vi "Email Handler (RT).vi"   [LabVIEW 2019]
types:
  T1 = cluster{"ArmedAddresses":i32[], "Tracker":i32, "EmailArray":i32[], "Armed":bool, "Inform":string, "Alarm":bool}
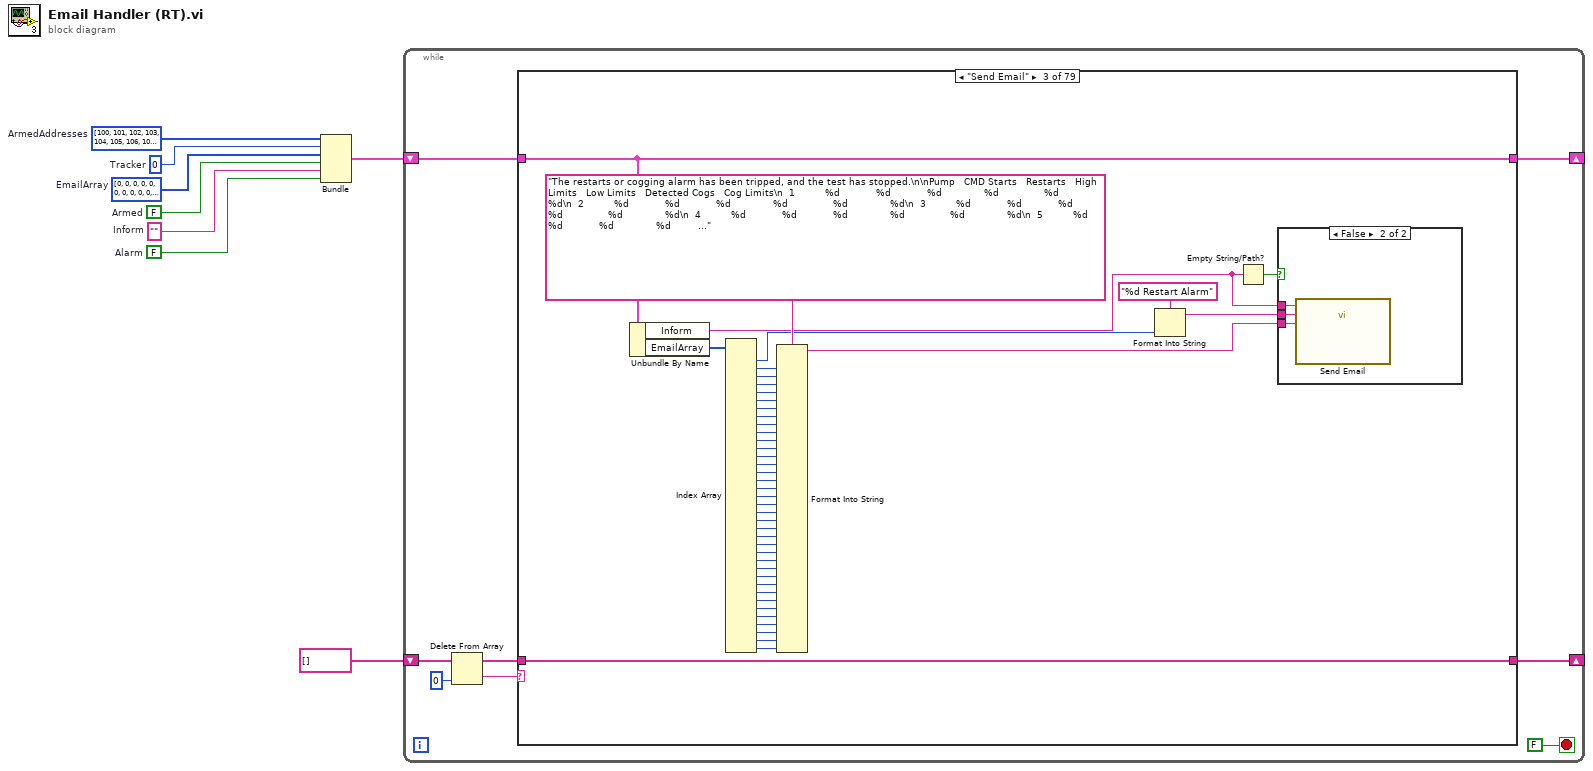
[diagram p0: block diagram]
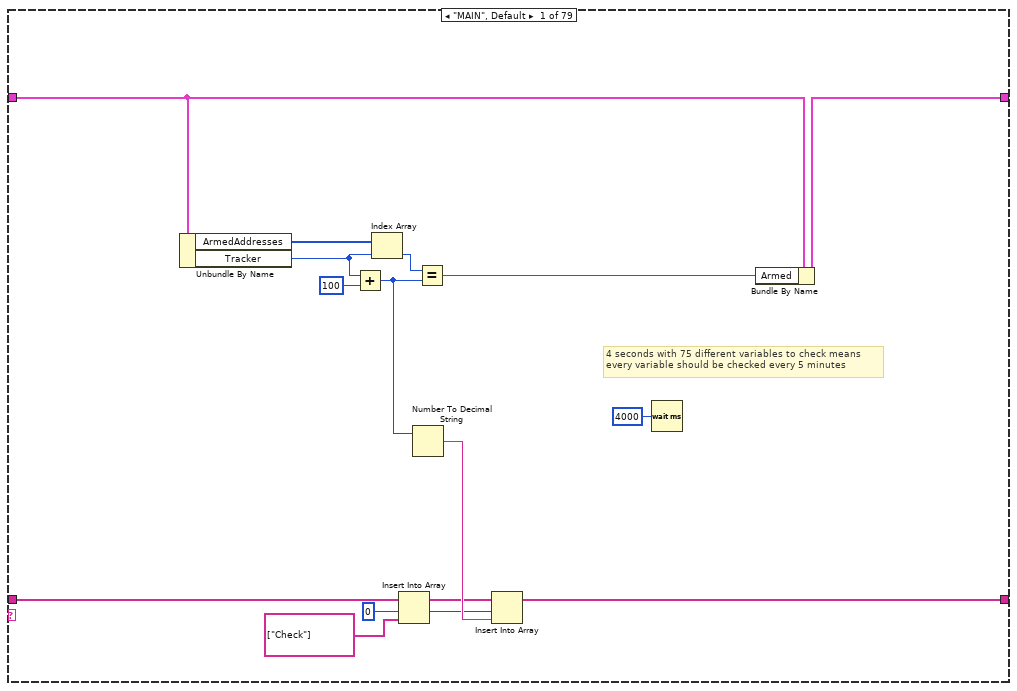
[diagram p2: hidden frame]
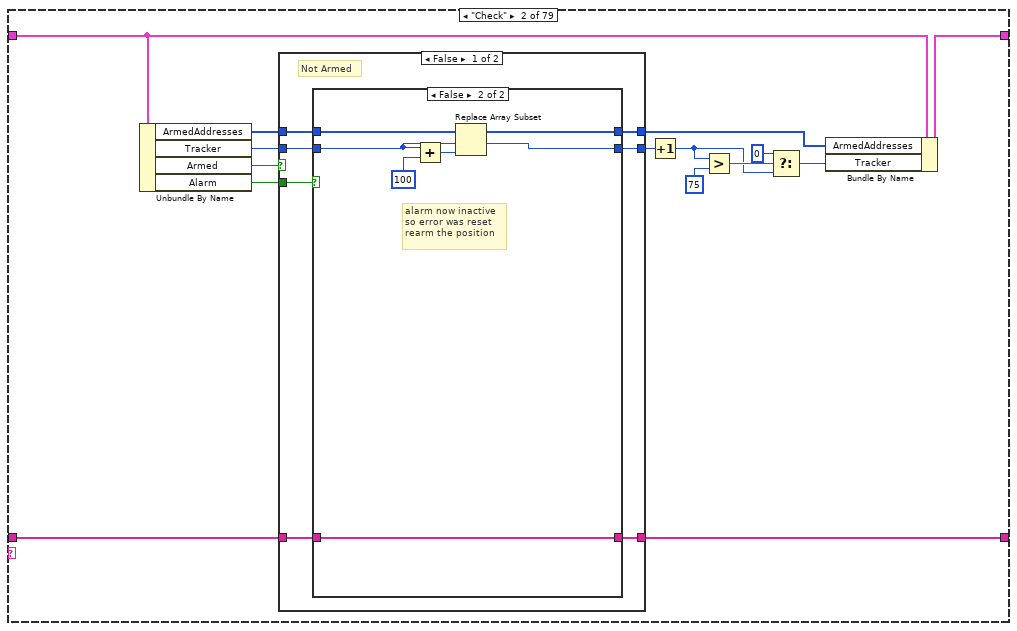
[diagram p3: hidden frame]
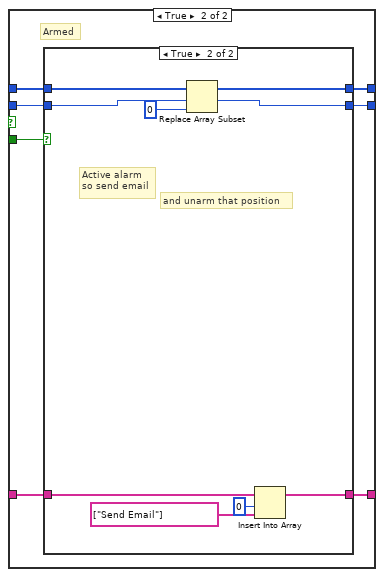
[diagram p5: hidden frame]
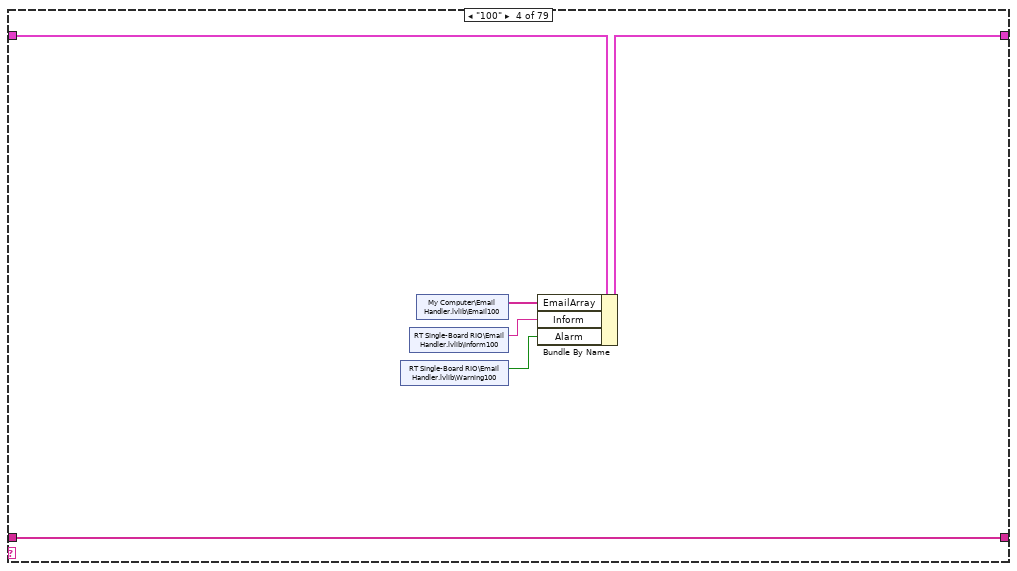
[diagram p8: hidden frame]
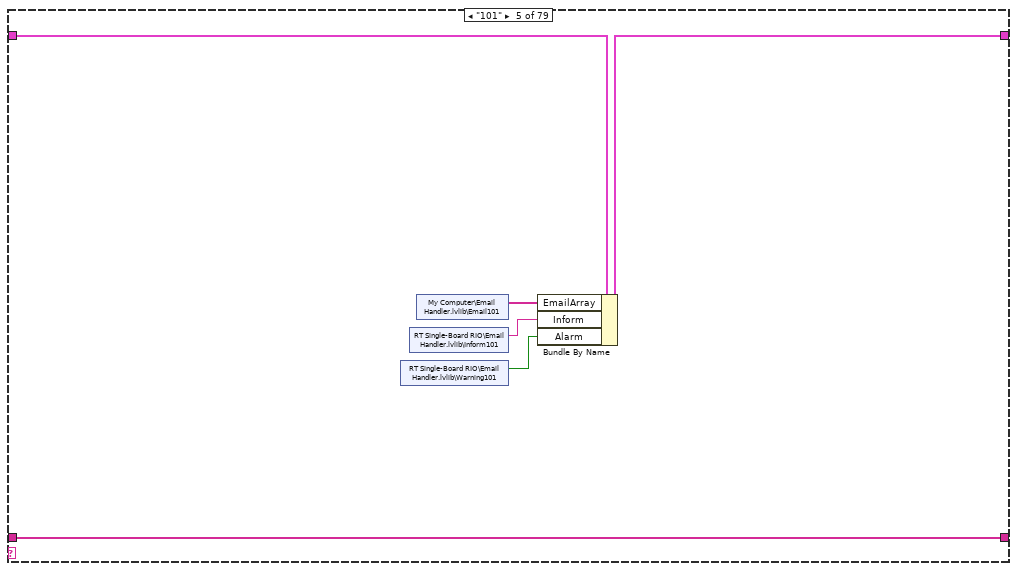
[diagram p9: hidden frame]
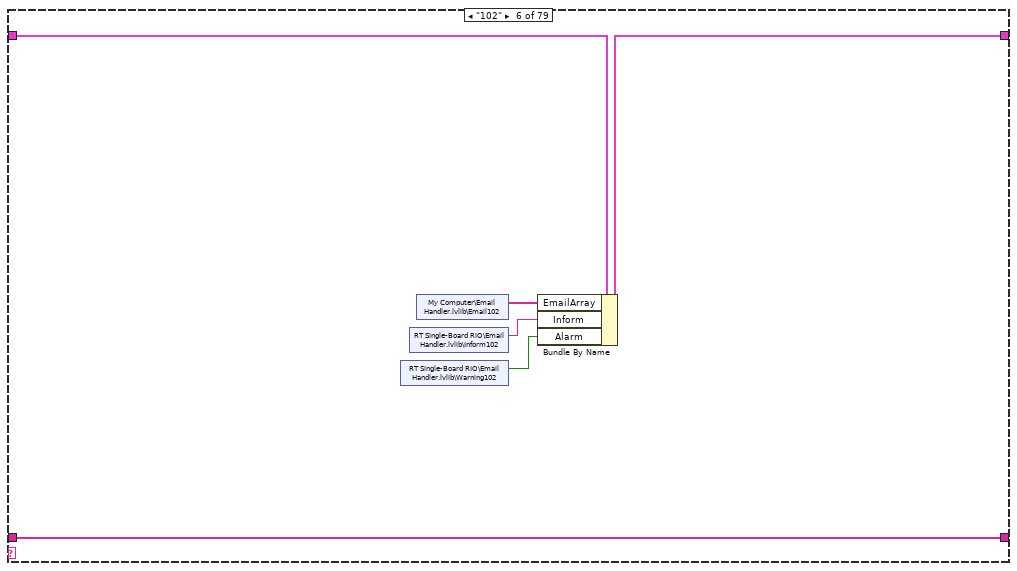
[diagram p10: hidden frame]
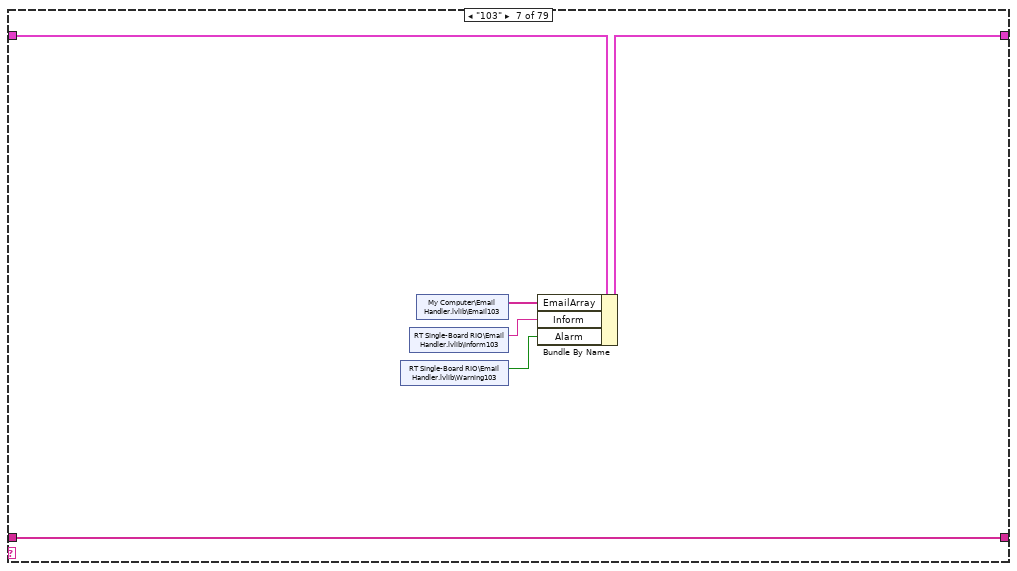
[diagram p11: hidden frame]
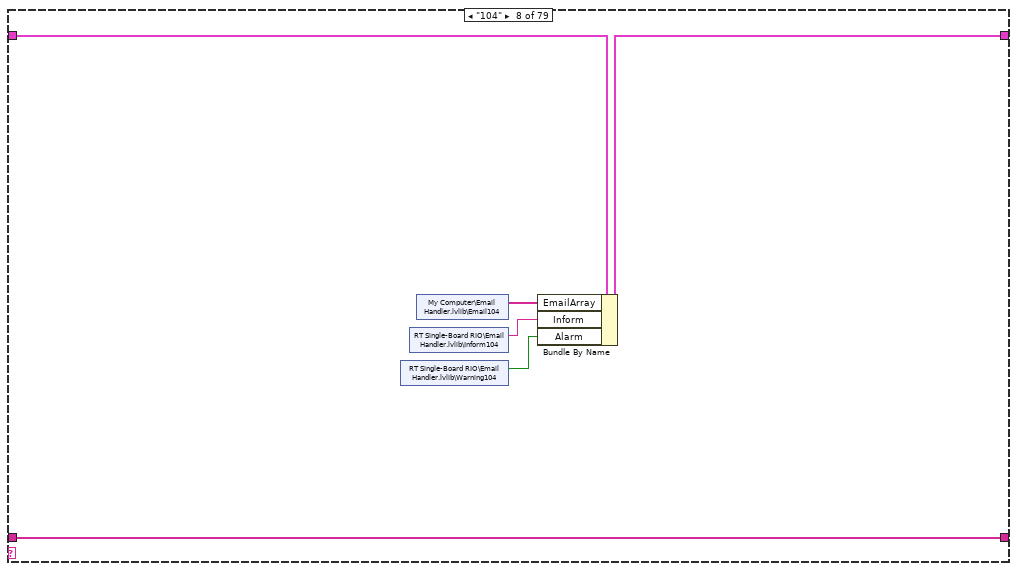
[diagram p12: hidden frame]
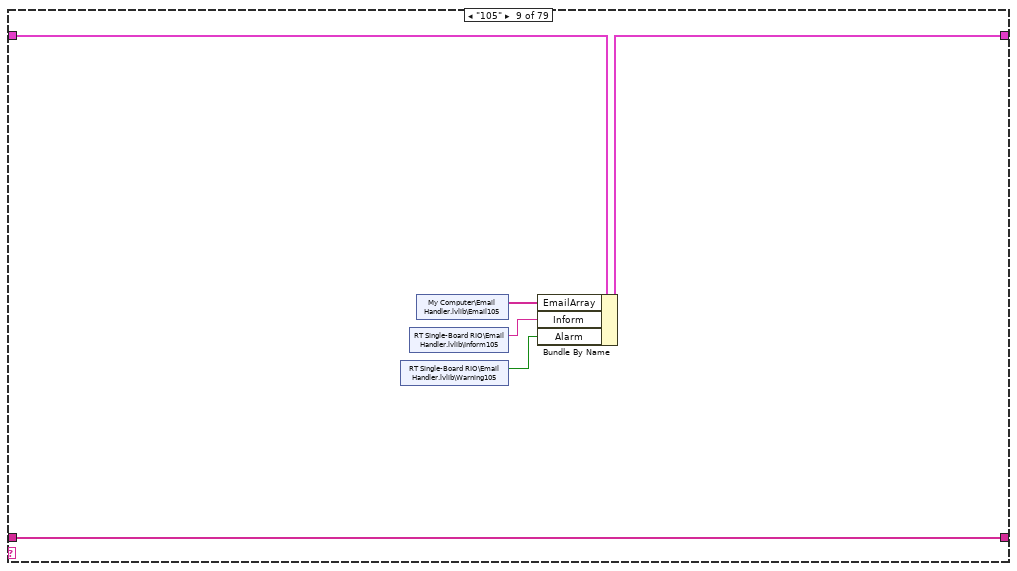
[diagram p13: hidden frame]
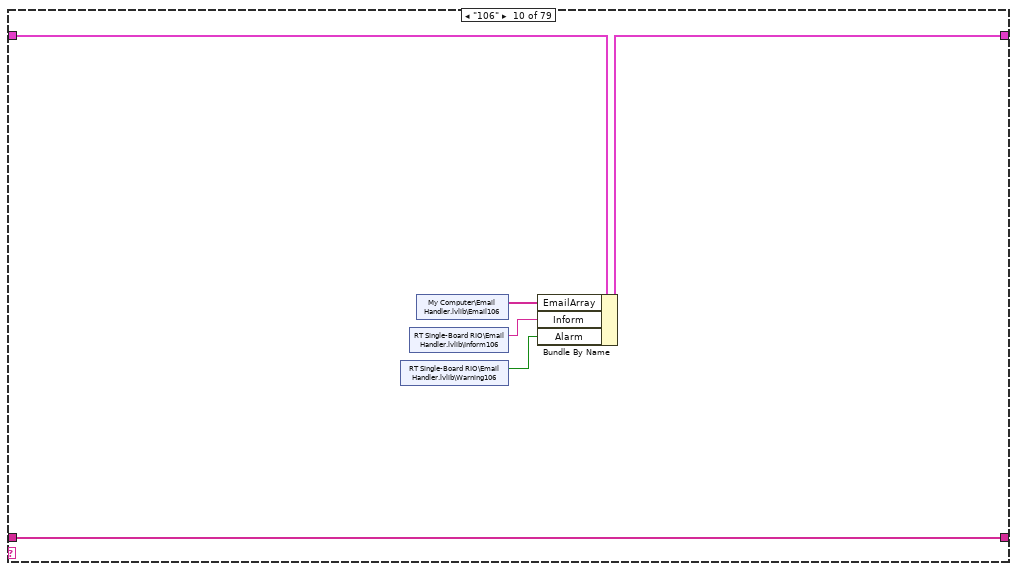
[diagram p14: hidden frame]
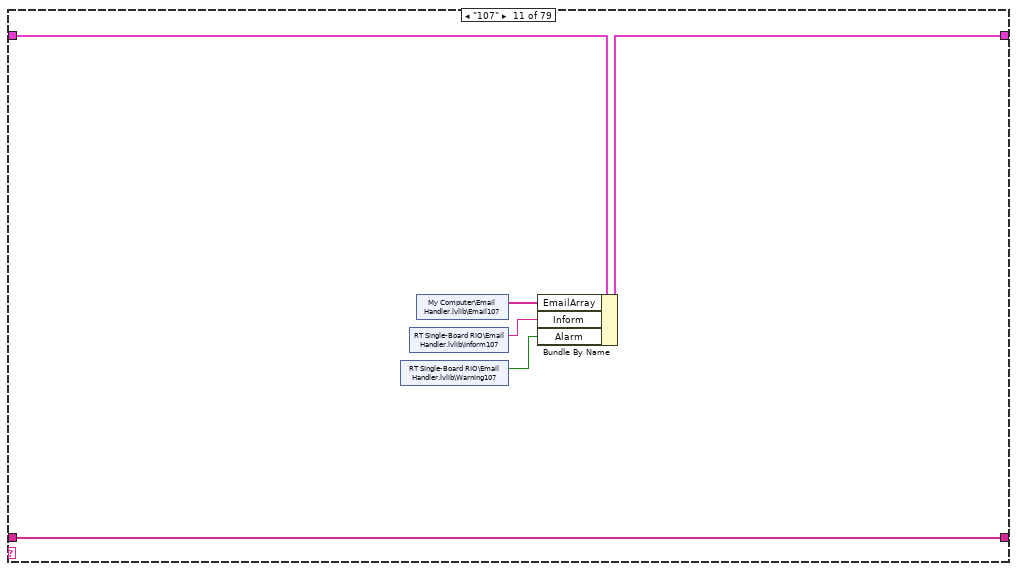
[diagram p15: hidden frame]
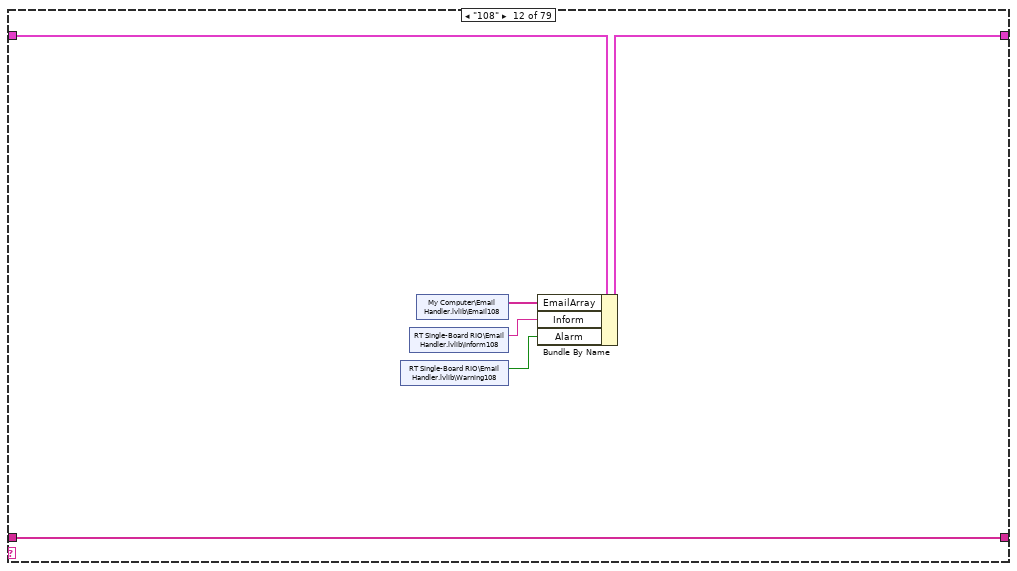
[diagram p16: hidden frame]
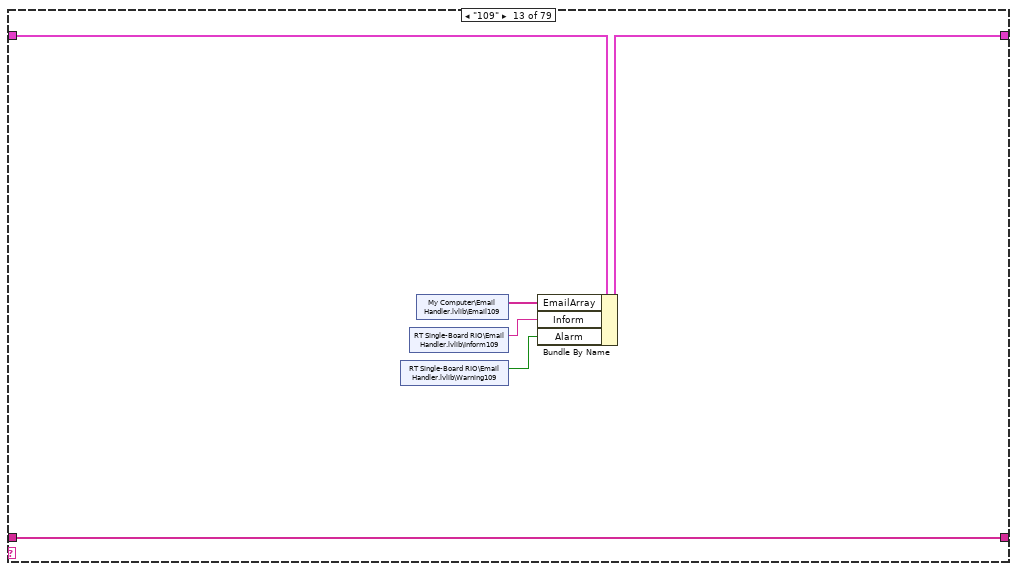
[diagram p17: hidden frame]
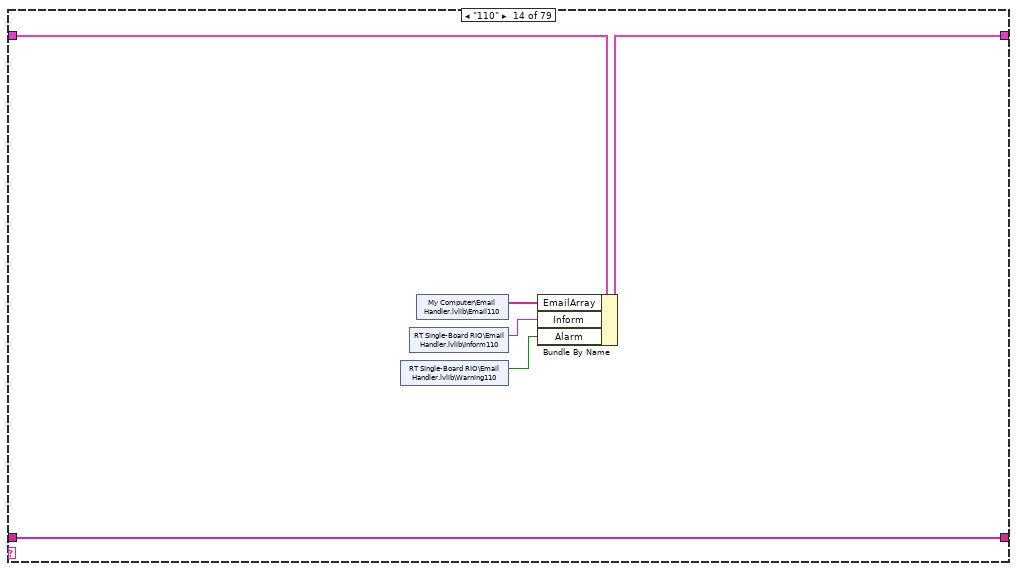
[diagram p18: hidden frame]
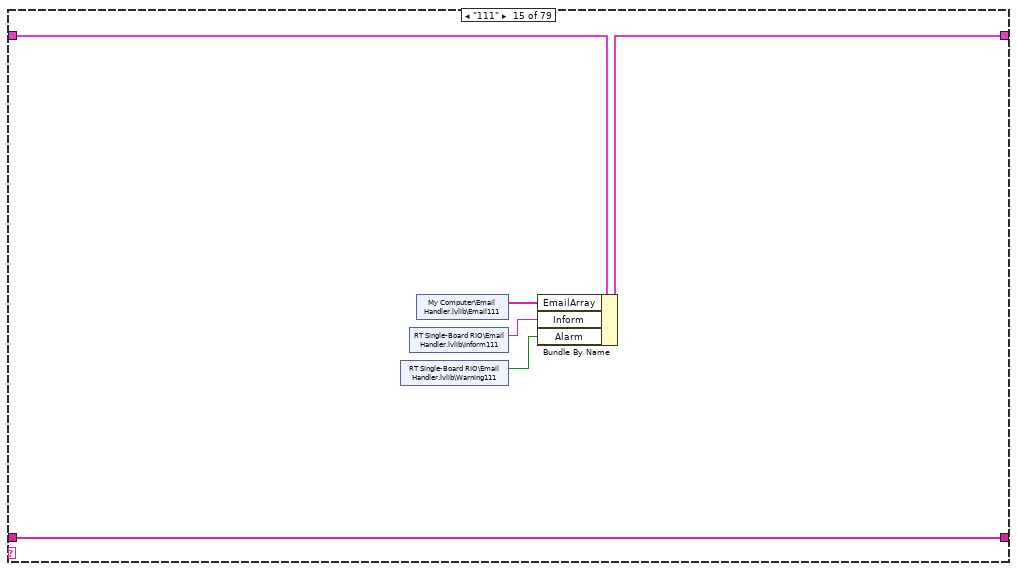
[diagram p19: hidden frame]
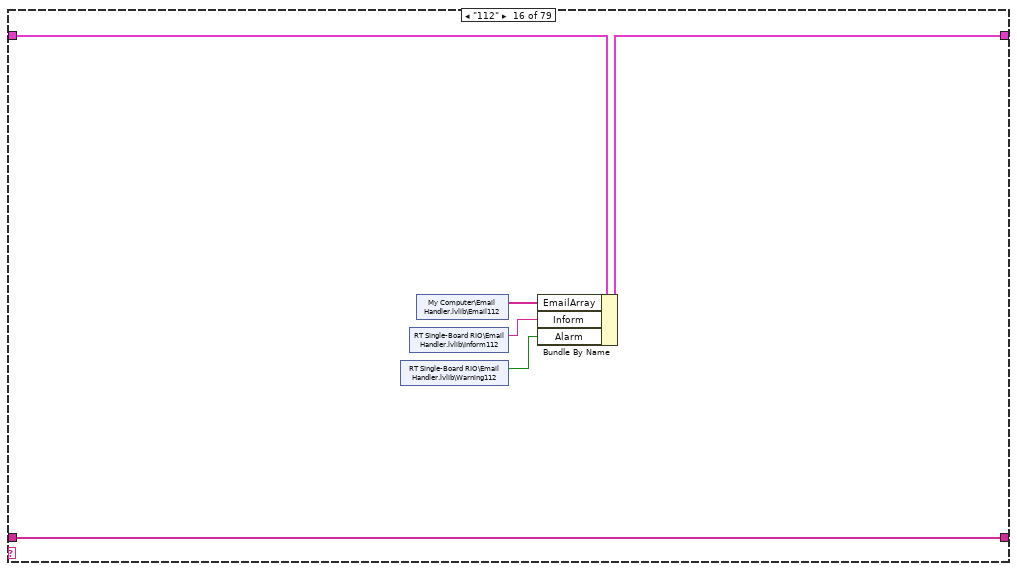
[diagram p20: hidden frame]
diagram:
  w1 = FALSE  # Alarm
  w2 = ""  # Inform
  w3 = FALSE  # Armed
  w4 = i32[] [0, 0, 0, 0, 0, 0, 0, 0, 0, 0, 0, 0, 0, 0, 0, 0, 0, 0, 0, 0, 0, 0, 0, 0, 0, 0, 0, 0, 0, 0, 0, 0, 0, 0, 0, 0, 0]  # EmailArray
  w6 = i32[] [100, 101, 102, 103, 104, 105, 106, 107, 108, 109, 110, 111, 112, 113, 114, 115, 116, 117, 118, 119, 120, 121, 122, 123, 124, 125, 126, 127, 128, 129, 130, 131, 132, 133, 134, 135, 136, 137, 138, 139, 140, 141, 142, 143, 144, 145, 146, 147, 148, 149, 150, 151, 152, 153, 154, 155, 156, 157, 158, 159, 160, 161, 162, 163, 164, 165, 166, 167, 168, 169, 170, 171, 172, 173, 174, 175]  # ArmedAddresses
  w8 = 0  # Tracker
  n1 = Bundle("ArmedAddresses"=w6, "Tracker"=w8, "EmailArray"=w4, "Armed"=w3, "Inform"=w2, "Alarm"=w1) -> (w7:T1)  [unwired: 1 in]
  n2 = while {
    shift-right: [w9] -> _
    shift-left: w7 -> [w15]
    shift-right: [w10] -> _
    shift-left: string[] [] -> [w14]
    stop <- FALSE stop-if-true
    n3 = Delete From Array(array=w14, index=0) -> (deleted portion=w12:string, array with subset deleted=w11:string[])  [unwired: 1 in]
    n4 = case shown="\"Send Email\"" w12 {
      tunnel: w15 -> [w29 w41 w125 w134 w140 w146 w152 w158 w164 w170 w176 w182 w188 w194 w200 w206 w212 w218 w224 w230 w236 w242 w248 w254 w260 w266 w272 w278 w284 w290 w296 w302 w308 w314 w320 w326 w332 w338 w344 w350 w356 w362 w368 w374 w380 w386 w392 w398 w404 w410 w416 w422 w428 w434 w440 w446 w452 w458 w464 w470 w476 w482 w488 w494 w500 w506 w512 w518 w524 w530 w536 w542 w548 w554 w560 w566 w572 w578 w584]
      tunnel: w11 -> [w21 w38 w126 w135 w141 w147 w153 w159 w165 w171 w177 w183 w189 w195 w201 w207 w213 w219 w225 w231 w237 w243 w249 w255 w261 w267 w273 w279 w285 w291 w297 w303 w309 w315 w321 w327 w333 w339 w345 w351 w357 w363 w369 w375 w381 w387 w393 w399 w405 w411 w417 w423 w429 w435 w441 w447 w453 w459 w465 w471 w477 w483 w489 w495 w501 w507 w513 w519 w525 w531 w537 w543 w549 w555 w561 w567 w573 w579 w585]
      tunnel: [w23 w35 w126 w135 w141 w147 w153 w159 w165 w171 w177 w183 w189 w195 w201 w207 w213 w219 w225 w231 w237 w243 w249 w255 w261 w267 w273 w279 w285 w291 w297 w303 w309 w315 w321 w327 w333 w339 w345 w351 w357 w363 w369 w375 w381 w387 w393 w399 w405 w411 w417 w423 w429 w435 w441 w447 w453 w459 w465 w471 w477 w483 w489 w495 w501 w507 w513 w519 w525 w531 w537 w543 w549 w555 w561 w567 w573 w579 w585] -> w10
      tunnel: [w28 w40 w125 w133 w139 w145 w151 w157 w163 w169 w175 w181 w187 w193 w199 w205 w211 w217 w223 w229 w235 w241 w247 w253 w259 w265 w271 w277 w283 w289 w295 w301 w307 w313 w319 w325 w331 w337 w343 w349 w355 w361 w367 w373 w379 w385 w391 w397 w403 w409 w415 w421 w427 w433 w439 w445 w451 w457 w463 w469 w475 w481 w487 w493 w499 w505 w511 w517 w523 w529 w535 w541 w547 w553 w559 w565 w571 w577 w583] -> w9
      frame "MAIN", Default {
        w19 = 0 ("index")
        # "4 seconds with 75 different variables to check means\nevery variable should be checked every 5 minutes"
        n5 = Unbundle By Name(w29) -> ("ArmedAddresses"=w30:i32[], "Tracker"=w17:i32)
        n6 = Add(x=w17, y=100) -> (x+y=w25:i32)
        n7 = Index Array(array=w30, index=w17) -> (element=w26:i32)
        n8 = Insert Into Array(array=w21, index=w19, new element=string[] ["Check"]) -> (w20:string[])
        n9 = Number To Decimal String(number=w25) -> (decimal integer string=w24:string)  [unwired: 1 in]
        n10 = Equal?(x=w26, y=w25) -> (x = y?=w22:bool)
        n11 = Insert Into Array(array=w20, index=w19, new element=w24) -> (w23:string[])
        n12 = Wait (ms)(milliseconds to wait=u32 4000) -> ()  [unwired: 1 out]
        n13 = Bundle By Name(cluster=w29, "Armed"=w22) -> (w28:T1)
      }
      frame "Check" {
        n14 = Unbundle By Name(w41) -> ("ArmedAddresses"=w34:i32[], "Tracker"=w37:i32, "Armed"=w39:bool, "Alarm"=w32:bool)
        n15 = case shown="False" w39 {
          tunnel: w38 -> [w53 w69]
          tunnel: w37 -> [w50 w66]
          tunnel: [w47 w63] -> w36
          tunnel: w32 -> [w49 w67]
          tunnel: [w52 w68] -> w35
          tunnel: w34 -> [w51 w65]
          tunnel: [w48 w64] -> w33
          frame False {
            # "Not Armed"
            n16 = case shown="False" w49 {
              tunnel: w53 -> [w54 w57]
              tunnel: [w54 w57] -> w52
              tunnel: w50 -> [w55 w60]
              tunnel: w51 -> [w56 w62]
              tunnel: [w56 w61] -> w48
              tunnel: [w55 w60] -> w47
              frame True {
                # "Alarm still active\nerror has not been reset\nleave unarmed"
              }
              frame False {
                # "alarm now inactive\nso error was reset\nrearm the position"
                n17 = Add(x=w60, y=100) -> (x+y=w59:i32)
                n18 = Replace Array Subset(array=w62, new element=w59, index=w60) -> (w61:i32[])
              }
            }
          }
          frame True {
            # "Armed"
            n19 = case shown="True" w67 {
              tunnel: w69 -> [w70 w80]
              tunnel: [w70 w79] -> w68
              tunnel: w66 -> [w71 w74]
              tunnel: w65 -> [w72 w76]
              tunnel: [w72 w75] -> w64
              tunnel: [w71 w74] -> w63
              frame False {
                # "No Alarm"
              }
              frame True {
                # "and unarm that position"
                # "Active alarm\nso send email"
                n20 = Replace Array Subset(array=w76, new element=0, index=w74) -> (w75:i32[])
                n21 = Insert Into Array(array=w80, index=0, new element=string[] ["Send Email"]) -> (w79:string[])
              }
            }
          }
        }
        n22 = Increment(x=w36) -> (x+1=w43:i32)
        n23 = Greater?(x=w43, y=75) -> (0:w45:bool)
        n24 = Select(t=0, s=w45, f=w43) -> (s? t:f=w42:i32)
        n25 = Bundle By Name(cluster=w41, "ArmedAddresses"=w33, "Tracker"=w42) -> (w40:T1)
      }
      frame "Send Email" {
        n26 = Unbundle By Name(w125) -> ("Inform"=w82:string, "EmailArray"=w96:i32[])
        n27 = Index Array(array=w96) -> (element #1=w83:i32, element #2=w100:i32, element #3=w101:i32, element #4=w102:i32, element #5=w103:i32, element #6=w104:i32, element #7=w105:i32, element #8=w106:i32, element #9=w107:i32, element #10=w108:i32, element #11=w109:i32, element #12=w110:i32, element #13=w111:i32, element #14=w114:i32, element #15=w113:i32, element #16=w115:i32, element #17=w116:i32, element #18=w117:i32, element #19=w118:i32, element #20=w119:i32, element #21=w120:i32, element #22=w121:i32, element #23=w122:i32, element #24=w123:i32, element #25=w124:i32, element #26=w95:i32, element #27=w94:i32, element #28=w93:i32, element #29=w92:i32, element #30=w91:i32, element #31=w90:i32, element #32=w89:i32, element #33=w88:i32, element #34=w87:i32, element #35=w86:i32, element #36=w85:i32, element #37=w84:i32)  [unwired: 37 in]
        n28 = Format Into String(format string="The restarts or cogging alarm has been tripped, and the test has stopped.\n\nPump   CMD Starts   Restarts   High Limits   Low Limits   Detected Cogs   Cog Limits\n  1          %d            %d            %d              %d               %d              %d\n  2          %d            %d            %d              %d               %d              %d\n  3          %d            %d            %d              %d               %d              %d\n  4          %d            %d            %d              %d               %d              %d\n  5          %d            %d            %d              %d               %d              %d\n  6          %d            %d            %d              %d               %d              %d" ("Message"), w100, w101, w102, w103, w104, w105, w106, w107, w108, w109, w110, w111, w114, w113, w115, w116, w117, w118, w119, w120, w121, w122, w123, w124, w95, w94, w93, w92, w91, w90, w89, w88, w87, w86, w85, w84) -> (resulting string=w112:string)  [unwired: 2 in, 1 out]
        n29 = Format Into String(format string="%d Restart Alarm", w83) -> (resulting string=w98:string)  [unwired: 2 in, 1 out]
        n30 = Empty String/Path?(string/path=w82) -> (empty?=w81:bool)
        n31 = case shown="False" w81 {
          tunnel: w112 -> [_ w129]
          tunnel: w98 -> [_ w128]
          tunnel: w82 -> [_ w127]
          frame True {
          }
          frame False {
            n32 = call "Send Email"("Message"=w129, "Subject"=w128, "Recipients"=w127) -> ()  [unwired: 8 in, 1 out]
          }
        }
      }
      frame "100" {
        n33 = shared-variable "RT Single-Board RIO\\Email Handler.lvlib\\Warning100"() -> (w130:bool)  [unwired: 1 in, 1 out]
        n34 = shared-variable "RT Single-Board RIO\\Email Handler.lvlib\\Inform100"() -> (w131:string)  [unwired: 1 in, 1 out]
        n35 = shared-variable "My Computer\\Email Handler.lvlib\\Email100"() -> (w132:string[])  [unwired: 1 in, 1 out]
        n36 = Bundle By Name(cluster=w134, "EmailArray"=w132, "Inform"=w131, "Alarm"=w130) -> (w133:T1)
      }
      frame "101" {
        n37 = shared-variable "RT Single-Board RIO\\Email Handler.lvlib\\Warning101"() -> (w136:bool)  [unwired: 1 in, 1 out]
        n38 = shared-variable "RT Single-Board RIO\\Email Handler.lvlib\\Inform101"() -> (w137:string)  [unwired: 1 in, 1 out]
        n39 = shared-variable "My Computer\\Email Handler.lvlib\\Email101"() -> (w138:string[])  [unwired: 1 in, 1 out]
        n40 = Bundle By Name(cluster=w140, "EmailArray"=w138, "Inform"=w137, "Alarm"=w136) -> (w139:T1)
      }
      frame "102" {
        n41 = shared-variable "RT Single-Board RIO\\Email Handler.lvlib\\Warning102"() -> (w142:bool)  [unwired: 1 in, 1 out]
        n42 = shared-variable "RT Single-Board RIO\\Email Handler.lvlib\\Inform102"() -> (w143:string)  [unwired: 1 in, 1 out]
        n43 = shared-variable "My Computer\\Email Handler.lvlib\\Email102"() -> (w144:string[])  [unwired: 1 in, 1 out]
        n44 = Bundle By Name(cluster=w146, "EmailArray"=w144, "Inform"=w143, "Alarm"=w142) -> (w145:T1)
      }
      frame "103" {
        n45 = shared-variable "RT Single-Board RIO\\Email Handler.lvlib\\Warning103"() -> (w148:bool)  [unwired: 1 in, 1 out]
        n46 = shared-variable "RT Single-Board RIO\\Email Handler.lvlib\\Inform103"() -> (w149:string)  [unwired: 1 in, 1 out]
        n47 = shared-variable "My Computer\\Email Handler.lvlib\\Email103"() -> (w150:string[])  [unwired: 1 in, 1 out]
        n48 = Bundle By Name(cluster=w152, "EmailArray"=w150, "Inform"=w149, "Alarm"=w148) -> (w151:T1)
      }
      frame "104" {
        n49 = shared-variable "RT Single-Board RIO\\Email Handler.lvlib\\Warning104"() -> (w154:bool)  [unwired: 1 in, 1 out]
        n50 = shared-variable "RT Single-Board RIO\\Email Handler.lvlib\\Inform104"() -> (w155:string)  [unwired: 1 in, 1 out]
        n51 = shared-variable "My Computer\\Email Handler.lvlib\\Email104"() -> (w156:string[])  [unwired: 1 in, 1 out]
        n52 = Bundle By Name(cluster=w158, "EmailArray"=w156, "Inform"=w155, "Alarm"=w154) -> (w157:T1)
      }
      frame "105" {
        n53 = shared-variable "RT Single-Board RIO\\Email Handler.lvlib\\Warning105"() -> (w160:bool)  [unwired: 1 in, 1 out]
        n54 = shared-variable "RT Single-Board RIO\\Email Handler.lvlib\\Inform105"() -> (w161:string)  [unwired: 1 in, 1 out]
        n55 = shared-variable "My Computer\\Email Handler.lvlib\\Email105"() -> (w162:string[])  [unwired: 1 in, 1 out]
        n56 = Bundle By Name(cluster=w164, "EmailArray"=w162, "Inform"=w161, "Alarm"=w160) -> (w163:T1)
      }
      frame "106" {
        n57 = shared-variable "RT Single-Board RIO\\Email Handler.lvlib\\Warning106"() -> (w166:bool)  [unwired: 1 in, 1 out]
        n58 = shared-variable "RT Single-Board RIO\\Email Handler.lvlib\\Inform106"() -> (w167:string)  [unwired: 1 in, 1 out]
        n59 = shared-variable "My Computer\\Email Handler.lvlib\\Email106"() -> (w168:string[])  [unwired: 1 in, 1 out]
        n60 = Bundle By Name(cluster=w170, "EmailArray"=w168, "Inform"=w167, "Alarm"=w166) -> (w169:T1)
      }
      frame "107" {
        n61 = shared-variable "RT Single-Board RIO\\Email Handler.lvlib\\Warning107"() -> (w172:bool)  [unwired: 1 in, 1 out]
        n62 = shared-variable "RT Single-Board RIO\\Email Handler.lvlib\\Inform107"() -> (w173:string)  [unwired: 1 in, 1 out]
        n63 = shared-variable "My Computer\\Email Handler.lvlib\\Email107"() -> (w174:string[])  [unwired: 1 in, 1 out]
        n64 = Bundle By Name(cluster=w176, "EmailArray"=w174, "Inform"=w173, "Alarm"=w172) -> (w175:T1)
      }
      frame "108" {
        n65 = shared-variable "RT Single-Board RIO\\Email Handler.lvlib\\Warning108"() -> (w178:bool)  [unwired: 1 in, 1 out]
        n66 = shared-variable "RT Single-Board RIO\\Email Handler.lvlib\\Inform108"() -> (w179:string)  [unwired: 1 in, 1 out]
        n67 = shared-variable "My Computer\\Email Handler.lvlib\\Email108"() -> (w180:string[])  [unwired: 1 in, 1 out]
        n68 = Bundle By Name(cluster=w182, "EmailArray"=w180, "Inform"=w179, "Alarm"=w178) -> (w181:T1)
      }
      frame "109" {
        n69 = shared-variable "RT Single-Board RIO\\Email Handler.lvlib\\Warning109"() -> (w184:bool)  [unwired: 1 in, 1 out]
        n70 = shared-variable "RT Single-Board RIO\\Email Handler.lvlib\\Inform109"() -> (w185:string)  [unwired: 1 in, 1 out]
        n71 = shared-variable "My Computer\\Email Handler.lvlib\\Email109"() -> (w186:string[])  [unwired: 1 in, 1 out]
        n72 = Bundle By Name(cluster=w188, "EmailArray"=w186, "Inform"=w185, "Alarm"=w184) -> (w187:T1)
      }
      frame "110" {
        n73 = shared-variable "RT Single-Board RIO\\Email Handler.lvlib\\Warning110"() -> (w190:bool)  [unwired: 1 in, 1 out]
        n74 = shared-variable "RT Single-Board RIO\\Email Handler.lvlib\\Inform110"() -> (w191:string)  [unwired: 1 in, 1 out]
        n75 = shared-variable "My Computer\\Email Handler.lvlib\\Email110"() -> (w192:string[])  [unwired: 1 in, 1 out]
        n76 = Bundle By Name(cluster=w194, "EmailArray"=w192, "Inform"=w191, "Alarm"=w190) -> (w193:T1)
      }
      frame "111" {
        n77 = shared-variable "RT Single-Board RIO\\Email Handler.lvlib\\Warning111"() -> (w196:bool)  [unwired: 1 in, 1 out]
        n78 = shared-variable "RT Single-Board RIO\\Email Handler.lvlib\\Inform111"() -> (w197:string)  [unwired: 1 in, 1 out]
        n79 = shared-variable "My Computer\\Email Handler.lvlib\\Email111"() -> (w198:string[])  [unwired: 1 in, 1 out]
        n80 = Bundle By Name(cluster=w200, "EmailArray"=w198, "Inform"=w197, "Alarm"=w196) -> (w199:T1)
      }
      frame "112" {
        n81 = shared-variable "RT Single-Board RIO\\Email Handler.lvlib\\Warning112"() -> (w202:bool)  [unwired: 1 in, 1 out]
        n82 = shared-variable "RT Single-Board RIO\\Email Handler.lvlib\\Inform112"() -> (w203:string)  [unwired: 1 in, 1 out]
        n83 = shared-variable "My Computer\\Email Handler.lvlib\\Email112"() -> (w204:string[])  [unwired: 1 in, 1 out]
        n84 = Bundle By Name(cluster=w206, "EmailArray"=w204, "Inform"=w203, "Alarm"=w202) -> (w205:T1)
      }
      frame "113" {
        n85 = shared-variable "RT Single-Board RIO\\Email Handler.lvlib\\Warning113"() -> (w208:bool)  [unwired: 1 in, 1 out]
        n86 = shared-variable "RT Single-Board RIO\\Email Handler.lvlib\\Inform113"() -> (w209:string)  [unwired: 1 in, 1 out]
        n87 = shared-variable "My Computer\\Email Handler.lvlib\\Email113"() -> (w210:string[])  [unwired: 1 in, 1 out]
        n88 = Bundle By Name(cluster=w212, "EmailArray"=w210, "Inform"=w209, "Alarm"=w208) -> (w211:T1)
      }
      frame "114" {
        n89 = shared-variable "RT Single-Board RIO\\Email Handler.lvlib\\Warning114"() -> (w214:bool)  [unwired: 1 in, 1 out]
        n90 = shared-variable "RT Single-Board RIO\\Email Handler.lvlib\\Inform114"() -> (w215:string)  [unwired: 1 in, 1 out]
        n91 = shared-variable "My Computer\\Email Handler.lvlib\\Email114"() -> (w216:string[])  [unwired: 1 in, 1 out]
        n92 = Bundle By Name(cluster=w218, "EmailArray"=w216, "Inform"=w215, "Alarm"=w214) -> (w217:T1)
      }
      frame "115" {
        n93 = shared-variable "RT Single-Board RIO\\Email Handler.lvlib\\Warning115"() -> (w220:bool)  [unwired: 1 in, 1 out]
        n94 = shared-variable "RT Single-Board RIO\\Email Handler.lvlib\\Inform115"() -> (w221:string)  [unwired: 1 in, 1 out]
        n95 = shared-variable "My Computer\\Email Handler.lvlib\\Email115"() -> (w222:string[])  [unwired: 1 in, 1 out]
        n96 = Bundle By Name(cluster=w224, "EmailArray"=w222, "Inform"=w221, "Alarm"=w220) -> (w223:T1)
      }
      frame "116" {
        n97 = shared-variable "RT Single-Board RIO\\Email Handler.lvlib\\Warning116"() -> (w226:bool)  [unwired: 1 in, 1 out]
        n98 = shared-variable "RT Single-Board RIO\\Email Handler.lvlib\\Inform116"() -> (w227:string)  [unwired: 1 in, 1 out]
        n99 = shared-variable "My Computer\\Email Handler.lvlib\\Email116"() -> (w228:string[])  [unwired: 1 in, 1 out]
        n100 = Bundle By Name(cluster=w230, "EmailArray"=w228, "Inform"=w227, "Alarm"=w226) -> (w229:T1)
      }
      frame "117" {
        n101 = shared-variable "RT Single-Board RIO\\Email Handler.lvlib\\Warning117"() -> (w232:bool)  [unwired: 1 in, 1 out]
        n102 = shared-variable "RT Single-Board RIO\\Email Handler.lvlib\\Inform117"() -> (w233:string)  [unwired: 1 in, 1 out]
        n103 = shared-variable "My Computer\\Email Handler.lvlib\\Email117"() -> (w234:string[])  [unwired: 1 in, 1 out]
        n104 = Bundle By Name(cluster=w236, "EmailArray"=w234, "Inform"=w233, "Alarm"=w232) -> (w235:T1)
      }
      frame "118" {
        n105 = shared-variable "RT Single-Board RIO\\Email Handler.lvlib\\Warning118"() -> (w238:bool)  [unwired: 1 in, 1 out]
        n106 = shared-variable "RT Single-Board RIO\\Email Handler.lvlib\\Inform118"() -> (w239:string)  [unwired: 1 in, 1 out]
        n107 = shared-variable "My Computer\\Email Handler.lvlib\\Email118"() -> (w240:string[])  [unwired: 1 in, 1 out]
        n108 = Bundle By Name(cluster=w242, "EmailArray"=w240, "Inform"=w239, "Alarm"=w238) -> (w241:T1)
      }
      frame "119" {
        n109 = shared-variable "RT Single-Board RIO\\Email Handler.lvlib\\Warning119"() -> (w244:bool)  [unwired: 1 in, 1 out]
        n110 = shared-variable "RT Single-Board RIO\\Email Handler.lvlib\\Inform119"() -> (w245:string)  [unwired: 1 in, 1 out]
        n111 = shared-variable "My Computer\\Email Handler.lvlib\\Email119"() -> (w246:string[])  [unwired: 1 in, 1 out]
        n112 = Bundle By Name(cluster=w248, "EmailArray"=w246, "Inform"=w245, "Alarm"=w244) -> (w247:T1)
      }
      frame "120" {
        n113 = shared-variable "RT Single-Board RIO\\Email Handler.lvlib\\Warning120"() -> (w250:bool)  [unwired: 1 in, 1 out]
        n114 = shared-variable "RT Single-Board RIO\\Email Handler.lvlib\\Inform120"() -> (w251:string)  [unwired: 1 in, 1 out]
        n115 = shared-variable "My Computer\\Email Handler.lvlib\\Email120"() -> (w252:string[])  [unwired: 1 in, 1 out]
        n116 = Bundle By Name(cluster=w254, "EmailArray"=w252, "Inform"=w251, "Alarm"=w250) -> (w253:T1)
      }
      frame "121" {
        n117 = shared-variable "RT Single-Board RIO\\Email Handler.lvlib\\Warning121"() -> (w256:bool)  [unwired: 1 in, 1 out]
        n118 = shared-variable "RT Single-Board RIO\\Email Handler.lvlib\\Inform121"() -> (w257:string)  [unwired: 1 in, 1 out]
        n119 = shared-variable "My Computer\\Email Handler.lvlib\\Email121"() -> (w258:string[])  [unwired: 1 in, 1 out]
        n120 = Bundle By Name(cluster=w260, "EmailArray"=w258, "Inform"=w257, "Alarm"=w256) -> (w259:T1)
      }
      frame "122" {
        n121 = shared-variable "RT Single-Board RIO\\Email Handler.lvlib\\Warning122"() -> (w262:bool)  [unwired: 1 in, 1 out]
        n122 = shared-variable "RT Single-Board RIO\\Email Handler.lvlib\\Inform122"() -> (w263:string)  [unwired: 1 in, 1 out]
        n123 = shared-variable "My Computer\\Email Handler.lvlib\\Email122"() -> (w264:string[])  [unwired: 1 in, 1 out]
        n124 = Bundle By Name(cluster=w266, "EmailArray"=w264, "Inform"=w263, "Alarm"=w262) -> (w265:T1)
      }
      frame "123" {
        n125 = shared-variable "RT Single-Board RIO\\Email Handler.lvlib\\Warning123"() -> (w268:bool)  [unwired: 1 in, 1 out]
        n126 = shared-variable "RT Single-Board RIO\\Email Handler.lvlib\\Inform123"() -> (w269:string)  [unwired: 1 in, 1 out]
        n127 = shared-variable "My Computer\\Email Handler.lvlib\\Email123"() -> (w270:string[])  [unwired: 1 in, 1 out]
        n128 = Bundle By Name(cluster=w272, "EmailArray"=w270, "Inform"=w269, "Alarm"=w268) -> (w271:T1)
      }
      frame "124" {
        n129 = shared-variable "RT Single-Board RIO\\Email Handler.lvlib\\Warning124"() -> (w274:bool)  [unwired: 1 in, 1 out]
        n130 = shared-variable "RT Single-Board RIO\\Email Handler.lvlib\\Inform124"() -> (w275:string)  [unwired: 1 in, 1 out]
        n131 = shared-variable "My Computer\\Email Handler.lvlib\\Email124"() -> (w276:string[])  [unwired: 1 in, 1 out]
        n132 = Bundle By Name(cluster=w278, "EmailArray"=w276, "Inform"=w275, "Alarm"=w274) -> (w277:T1)
      }
      frame "125" {
        n133 = shared-variable "RT Single-Board RIO\\Email Handler.lvlib\\Warning125"() -> (w280:bool)  [unwired: 1 in, 1 out]
        n134 = shared-variable "RT Single-Board RIO\\Email Handler.lvlib\\Inform125"() -> (w281:string)  [unwired: 1 in, 1 out]
        n135 = shared-variable "My Computer\\Email Handler.lvlib\\Email125"() -> (w282:string[])  [unwired: 1 in, 1 out]
        n136 = Bundle By Name(cluster=w284, "EmailArray"=w282, "Inform"=w281, "Alarm"=w280) -> (w283:T1)
      }
      frame "126" {
        n137 = shared-variable "RT Single-Board RIO\\Email Handler.lvlib\\Warning126"() -> (w286:bool)  [unwired: 1 in, 1 out]
        n138 = shared-variable "RT Single-Board RIO\\Email Handler.lvlib\\Inform126"() -> (w287:string)  [unwired: 1 in, 1 out]
        n139 = shared-variable "My Computer\\Email Handler.lvlib\\Email126"() -> (w288:string[])  [unwired: 1 in, 1 out]
        n140 = Bundle By Name(cluster=w290, "EmailArray"=w288, "Inform"=w287, "Alarm"=w286) -> (w289:T1)
      }
      frame "127" {
        n141 = shared-variable "RT Single-Board RIO\\Email Handler.lvlib\\Warning127"() -> (w292:bool)  [unwired: 1 in, 1 out]
        n142 = shared-variable "RT Single-Board RIO\\Email Handler.lvlib\\Inform127"() -> (w293:string)  [unwired: 1 in, 1 out]
        n143 = shared-variable "My Computer\\Email Handler.lvlib\\Email127"() -> (w294:string[])  [unwired: 1 in, 1 out]
        n144 = Bundle By Name(cluster=w296, "EmailArray"=w294, "Inform"=w293, "Alarm"=w292) -> (w295:T1)
      }
      frame "128" {
        n145 = shared-variable "RT Single-Board RIO\\Email Handler.lvlib\\Warning128"() -> (w298:bool)  [unwired: 1 in, 1 out]
        n146 = shared-variable "RT Single-Board RIO\\Email Handler.lvlib\\Inform128"() -> (w299:string)  [unwired: 1 in, 1 out]
        n147 = shared-variable "My Computer\\Email Handler.lvlib\\Email128"() -> (w300:string[])  [unwired: 1 in, 1 out]
        n148 = Bundle By Name(cluster=w302, "EmailArray"=w300, "Inform"=w299, "Alarm"=w298) -> (w301:T1)
      }
      frame "129" {
        n149 = shared-variable "RT Single-Board RIO\\Email Handler.lvlib\\Warning129"() -> (w304:bool)  [unwired: 1 in, 1 out]
        n150 = shared-variable "RT Single-Board RIO\\Email Handler.lvlib\\Inform129"() -> (w305:string)  [unwired: 1 in, 1 out]
        n151 = shared-variable "My Computer\\Email Handler.lvlib\\Email129"() -> (w306:string[])  [unwired: 1 in, 1 out]
        n152 = Bundle By Name(cluster=w308, "EmailArray"=w306, "Inform"=w305, "Alarm"=w304) -> (w307:T1)
      }
      frame "130" {
        n153 = shared-variable "RT Single-Board RIO\\Email Handler.lvlib\\Warning130"() -> (w310:bool)  [unwired: 1 in, 1 out]
        n154 = shared-variable "RT Single-Board RIO\\Email Handler.lvlib\\Inform130"() -> (w311:string)  [unwired: 1 in, 1 out]
        n155 = shared-variable "My Computer\\Email Handler.lvlib\\Email130"() -> (w312:string[])  [unwired: 1 in, 1 out]
        n156 = Bundle By Name(cluster=w314, "EmailArray"=w312, "Inform"=w311, "Alarm"=w310) -> (w313:T1)
      }
      frame "131" {
        n157 = shared-variable "RT Single-Board RIO\\Email Handler.lvlib\\Warning131"() -> (w316:bool)  [unwired: 1 in, 1 out]
        n158 = shared-variable "RT Single-Board RIO\\Email Handler.lvlib\\Inform131"() -> (w317:string)  [unwired: 1 in, 1 out]
        n159 = shared-variable "My Computer\\Email Handler.lvlib\\Email131"() -> (w318:string[])  [unwired: 1 in, 1 out]
        n160 = Bundle By Name(cluster=w320, "EmailArray"=w318, "Inform"=w317, "Alarm"=w316) -> (w319:T1)
      }
      frame "132" {
        n161 = shared-variable "RT Single-Board RIO\\Email Handler.lvlib\\Warning132"() -> (w322:bool)  [unwired: 1 in, 1 out]
        n162 = shared-variable "RT Single-Board RIO\\Email Handler.lvlib\\Inform132"() -> (w323:string)  [unwired: 1 in, 1 out]
        n163 = shared-variable "My Computer\\Email Handler.lvlib\\Email132"() -> (w324:string[])  [unwired: 1 in, 1 out]
        n164 = Bundle By Name(cluster=w326, "EmailArray"=w324, "Inform"=w323, "Alarm"=w322) -> (w325:T1)
      }
      frame "133" {
        n165 = shared-variable "RT Single-Board RIO\\Email Handler.lvlib\\Warning133"() -> (w328:bool)  [unwired: 1 in, 1 out]
        n166 = shared-variable "RT Single-Board RIO\\Email Handler.lvlib\\Inform133"() -> (w329:string)  [unwired: 1 in, 1 out]
        n167 = shared-variable "My Computer\\Email Handler.lvlib\\Email133"() -> (w330:string[])  [unwired: 1 in, 1 out]
        n168 = Bundle By Name(cluster=w332, "EmailArray"=w330, "Inform"=w329, "Alarm"=w328) -> (w331:T1)
      }
      frame "134" {
        n169 = shared-variable "RT Single-Board RIO\\Email Handler.lvlib\\Warning134"() -> (w334:bool)  [unwired: 1 in, 1 out]
        n170 = shared-variable "RT Single-Board RIO\\Email Handler.lvlib\\Inform134"() -> (w335:string)  [unwired: 1 in, 1 out]
        n171 = shared-variable "My Computer\\Email Handler.lvlib\\Email134"() -> (w336:string[])  [unwired: 1 in, 1 out]
        n172 = Bundle By Name(cluster=w338, "EmailArray"=w336, "Inform"=w335, "Alarm"=w334) -> (w337:T1)
      }
      frame "135" {
        n173 = shared-variable "RT Single-Board RIO\\Email Handler.lvlib\\Warning135"() -> (w340:bool)  [unwired: 1 in, 1 out]
        n174 = shared-variable "RT Single-Board RIO\\Email Handler.lvlib\\Inform135"() -> (w341:string)  [unwired: 1 in, 1 out]
        n175 = shared-variable "My Computer\\Email Handler.lvlib\\Email135"() -> (w342:string[])  [unwired: 1 in, 1 out]
        n176 = Bundle By Name(cluster=w344, "EmailArray"=w342, "Inform"=w341, "Alarm"=w340) -> (w343:T1)
      }
      frame "136" {
        n177 = shared-variable "RT Single-Board RIO\\Email Handler.lvlib\\Warning136"() -> (w346:bool)  [unwired: 1 in, 1 out]
        n178 = shared-variable "RT Single-Board RIO\\Email Handler.lvlib\\Inform136"() -> (w347:string)  [unwired: 1 in, 1 out]
        n179 = shared-variable "My Computer\\Email Handler.lvlib\\Email136"() -> (w348:string[])  [unwired: 1 in, 1 out]
        n180 = Bundle By Name(cluster=w350, "EmailArray"=w348, "Inform"=w347, "Alarm"=w346) -> (w349:T1)
      }
      frame "137" {
        n181 = shared-variable "RT Single-Board RIO\\Email Handler.lvlib\\Warning137"() -> (w352:bool)  [unwired: 1 in, 1 out]
        n182 = shared-variable "RT Single-Board RIO\\Email Handler.lvlib\\Inform137"() -> (w353:string)  [unwired: 1 in, 1 out]
        n183 = shared-variable "My Computer\\Email Handler.lvlib\\Email137"() -> (w354:string[])  [unwired: 1 in, 1 out]
        n184 = Bundle By Name(cluster=w356, "EmailArray"=w354, "Inform"=w353, "Alarm"=w352) -> (w355:T1)
      }
      frame "138" {
        n185 = shared-variable "RT Single-Board RIO\\Email Handler.lvlib\\Warning138"() -> (w358:bool)  [unwired: 1 in, 1 out]
        n186 = shared-variable "RT Single-Board RIO\\Email Handler.lvlib\\Inform138"() -> (w359:string)  [unwired: 1 in, 1 out]
        n187 = shared-variable "My Computer\\Email Handler.lvlib\\Email138"() -> (w360:string[])  [unwired: 1 in, 1 out]
        n188 = Bundle By Name(cluster=w362, "EmailArray"=w360, "Inform"=w359, "Alarm"=w358) -> (w361:T1)
      }
      frame "139" {
        n189 = shared-variable "RT Single-Board RIO\\Email Handler.lvlib\\Warning139"() -> (w364:bool)  [unwired: 1 in, 1 out]
        n190 = shared-variable "RT Single-Board RIO\\Email Handler.lvlib\\Inform139"() -> (w365:string)  [unwired: 1 in, 1 out]
        n191 = shared-variable "My Computer\\Email Handler.lvlib\\Email139"() -> (w366:string[])  [unwired: 1 in, 1 out]
        n192 = Bundle By Name(cluster=w368, "EmailArray"=w366, "Inform"=w365, "Alarm"=w364) -> (w367:T1)
      }
      frame "140" {
        n193 = shared-variable "RT Single-Board RIO\\Email Handler.lvlib\\Warning140"() -> (w370:bool)  [unwired: 1 in, 1 out]
        n194 = shared-variable "RT Single-Board RIO\\Email Handler.lvlib\\Inform140"() -> (w371:string)  [unwired: 1 in, 1 out]
        n195 = shared-variable "My Computer\\Email Handler.lvlib\\Email140"() -> (w372:string[])  [unwired: 1 in, 1 out]
        n196 = Bundle By Name(cluster=w374, "EmailArray"=w372, "Inform"=w371, "Alarm"=w370) -> (w373:T1)
      }
      frame "141" {
        n197 = shared-variable "RT Single-Board RIO\\Email Handler.lvlib\\Warning141"() -> (w376:bool)  [unwired: 1 in, 1 out]
        n198 = shared-variable "RT Single-Board RIO\\Email Handler.lvlib\\Inform141"() -> (w377:string)  [unwired: 1 in, 1 out]
        n199 = shared-variable "My Computer\\Email Handler.lvlib\\Email141"() -> (w378:string[])  [unwired: 1 in, 1 out]
        n200 = Bundle By Name(cluster=w380, "EmailArray"=w378, "Inform"=w377, "Alarm"=w376) -> (w379:T1)
      }
      frame "142" {
        n201 = shared-variable "RT Single-Board RIO\\Email Handler.lvlib\\Warning142"() -> (w382:bool)  [unwired: 1 in, 1 out]
        n202 = shared-variable "RT Single-Board RIO\\Email Handler.lvlib\\Inform142"() -> (w383:string)  [unwired: 1 in, 1 out]
        n203 = shared-variable "My Computer\\Email Handler.lvlib\\Email142"() -> (w384:string[])  [unwired: 1 in, 1 out]
        n204 = Bundle By Name(cluster=w386, "EmailArray"=w384, "Inform"=w383, "Alarm"=w382) -> (w385:T1)
      }
      frame "143" {
        n205 = shared-variable "RT Single-Board RIO\\Email Handler.lvlib\\Warning143"() -> (w388:bool)  [unwired: 1 in, 1 out]
        n206 = shared-variable "RT Single-Board RIO\\Email Handler.lvlib\\Inform143"() -> (w389:string)  [unwired: 1 in, 1 out]
        n207 = shared-variable "My Computer\\Email Handler.lvlib\\Email143"() -> (w390:string[])  [unwired: 1 in, 1 out]
        n208 = Bundle By Name(cluster=w392, "EmailArray"=w390, "Inform"=w389, "Alarm"=w388) -> (w391:T1)
      }
      frame "144" {
        n209 = shared-variable "RT Single-Board RIO\\Email Handler.lvlib\\Warning144"() -> (w394:bool)  [unwired: 1 in, 1 out]
        n210 = shared-variable "RT Single-Board RIO\\Email Handler.lvlib\\Inform144"() -> (w395:string)  [unwired: 1 in, 1 out]
        n211 = shared-variable "My Computer\\Email Handler.lvlib\\Email144"() -> (w396:string[])  [unwired: 1 in, 1 out]
        n212 = Bundle By Name(cluster=w398, "EmailArray"=w396, "Inform"=w395, "Alarm"=w394) -> (w397:T1)
      }
      frame "145" {
        n213 = shared-variable "RT Single-Board RIO\\Email Handler.lvlib\\Warning145"() -> (w400:bool)  [unwired: 1 in, 1 out]
        n214 = shared-variable "RT Single-Board RIO\\Email Handler.lvlib\\Inform145"() -> (w401:string)  [unwired: 1 in, 1 out]
        n215 = shared-variable "My Computer\\Email Handler.lvlib\\Email145"() -> (w402:string[])  [unwired: 1 in, 1 out]
        n216 = Bundle By Name(cluster=w404, "EmailArray"=w402, "Inform"=w401, "Alarm"=w400) -> (w403:T1)
      }
      frame "146" {
        n217 = shared-variable "RT Single-Board RIO\\Email Handler.lvlib\\Warning146"() -> (w406:bool)  [unwired: 1 in, 1 out]
        n218 = shared-variable "RT Single-Board RIO\\Email Handler.lvlib\\Inform146"() -> (w407:string)  [unwired: 1 in, 1 out]
        n219 = shared-variable "My Computer\\Email Handler.lvlib\\Email146"() -> (w408:string[])  [unwired: 1 in, 1 out]
        n220 = Bundle By Name(cluster=w410, "EmailArray"=w408, "Inform"=w407, "Alarm"=w406) -> (w409:T1)
      }
      frame "147" {
        n221 = shared-variable "RT Single-Board RIO\\Email Handler.lvlib\\Warning147"() -> (w412:bool)  [unwired: 1 in, 1 out]
        n222 = shared-variable "RT Single-Board RIO\\Email Handler.lvlib\\Inform147"() -> (w413:string)  [unwired: 1 in, 1 out]
        n223 = shared-variable "My Computer\\Email Handler.lvlib\\Email147"() -> (w414:string[])  [unwired: 1 in, 1 out]
        n224 = Bundle By Name(cluster=w416, "EmailArray"=w414, "Inform"=w413, "Alarm"=w412) -> (w415:T1)
      }
      frame "148" {
        n225 = shared-variable "RT Single-Board RIO\\Email Handler.lvlib\\Warning148"() -> (w418:bool)  [unwired: 1 in, 1 out]
        n226 = shared-variable "RT Single-Board RIO\\Email Handler.lvlib\\Inform148"() -> (w419:string)  [unwired: 1 in, 1 out]
        n227 = shared-variable "My Computer\\Email Handler.lvlib\\Email148"() -> (w420:string[])  [unwired: 1 in, 1 out]
        n228 = Bundle By Name(cluster=w422, "EmailArray"=w420, "Inform"=w419, "Alarm"=w418) -> (w421:T1)
      }
      frame "149" {
        n229 = shared-variable "RT Single-Board RIO\\Email Handler.lvlib\\Warning149"() -> (w424:bool)  [unwired: 1 in, 1 out]
        n230 = shared-variable "RT Single-Board RIO\\Email Handler.lvlib\\Inform149"() -> (w425:string)  [unwired: 1 in, 1 out]
        n231 = shared-variable "My Computer\\Email Handler.lvlib\\Email149"() -> (w426:string[])  [unwired: 1 in, 1 out]
        n232 = Bundle By Name(cluster=w428, "EmailArray"=w426, "Inform"=w425, "Alarm"=w424) -> (w427:T1)
      }
      frame "150" {
        n233 = shared-variable "RT Single-Board RIO\\Email Handler.lvlib\\Warning150"() -> (w430:bool)  [unwired: 1 in, 1 out]
        n234 = shared-variable "RT Single-Board RIO\\Email Handler.lvlib\\Inform150"() -> (w431:string)  [unwired: 1 in, 1 out]
        n235 = shared-variable "My Computer\\Email Handler.lvlib\\Email150"() -> (w432:string[])  [unwired: 1 in, 1 out]
        n236 = Bundle By Name(cluster=w434, "EmailArray"=w432, "Inform"=w431, "Alarm"=w430) -> (w433:T1)
      }
      frame "151" {
        n237 = shared-variable "RT Single-Board RIO\\Email Handler.lvlib\\Warning151"() -> (w436:bool)  [unwired: 1 in, 1 out]
        n238 = shared-variable "RT Single-Board RIO\\Email Handler.lvlib\\Inform151"() -> (w437:string)  [unwired: 1 in, 1 out]
        n239 = shared-variable "My Computer\\Email Handler.lvlib\\Email151"() -> (w438:string[])  [unwired: 1 in, 1 out]
        n240 = Bundle By Name(cluster=w440, "EmailArray"=w438, "Inform"=w437, "Alarm"=w436) -> (w439:T1)
      }
      frame "152" {
        n241 = shared-variable "RT Single-Board RIO\\Email Handler.lvlib\\Warning152"() -> (w442:bool)  [unwired: 1 in, 1 out]
        n242 = shared-variable "RT Single-Board RIO\\Email Handler.lvlib\\Inform152"() -> (w443:string)  [unwired: 1 in, 1 out]
        n243 = shared-variable "My Computer\\Email Handler.lvlib\\Email152"() -> (w444:string[])  [unwired: 1 in, 1 out]
        n244 = Bundle By Name(cluster=w446, "EmailArray"=w444, "Inform"=w443, "Alarm"=w442) -> (w445:T1)
      }
      frame "153" {
        n245 = shared-variable "RT Single-Board RIO\\Email Handler.lvlib\\Warning153"() -> (w448:bool)  [unwired: 1 in, 1 out]
        n246 = shared-variable "RT Single-Board RIO\\Email Handler.lvlib\\Inform153"() -> (w449:string)  [unwired: 1 in, 1 out]
        n247 = shared-variable "My Computer\\Email Handler.lvlib\\Email153"() -> (w450:string[])  [unwired: 1 in, 1 out]
        n248 = Bundle By Name(cluster=w452, "EmailArray"=w450, "Inform"=w449, "Alarm"=w448) -> (w451:T1)
      }
      frame "154" {
        n249 = shared-variable "RT Single-Board RIO\\Email Handler.lvlib\\Warning154"() -> (w454:bool)  [unwired: 1 in, 1 out]
        n250 = shared-variable "RT Single-Board RIO\\Email Handler.lvlib\\Inform154"() -> (w455:string)  [unwired: 1 in, 1 out]
        n251 = shared-variable "My Computer\\Email Handler.lvlib\\Email154"() -> (w456:string[])  [unwired: 1 in, 1 out]
        n252 = Bundle By Name(cluster=w458, "EmailArray"=w456, "Inform"=w455, "Alarm"=w454) -> (w457:T1)
      }
      frame "155" {
        n253 = shared-variable "RT Single-Board RIO\\Email Handler.lvlib\\Warning155"() -> (w460:bool)  [unwired: 1 in, 1 out]
        n254 = shared-variable "RT Single-Board RIO\\Email Handler.lvlib\\Inform155"() -> (w461:string)  [unwired: 1 in, 1 out]
        n255 = shared-variable "My Computer\\Email Handler.lvlib\\Email155"() -> (w462:string[])  [unwired: 1 in, 1 out]
        n256 = Bundle By Name(cluster=w464, "EmailArray"=w462, "Inform"=w461, "Alarm"=w460) -> (w463:T1)
      }
      frame "156" {
        n257 = shared-variable "RT Single-Board RIO\\Email Handler.lvlib\\Warning156"() -> (w466:bool)  [unwired: 1 in, 1 out]
        n258 = shared-variable "RT Single-Board RIO\\Email Handler.lvlib\\Inform156"() -> (w467:string)  [unwired: 1 in, 1 out]
        n259 = shared-variable "My Computer\\Email Handler.lvlib\\Email156"() -> (w468:string[])  [unwired: 1 in, 1 out]
        n260 = Bundle By Name(cluster=w470, "EmailArray"=w468, "Inform"=w467, "Alarm"=w466) -> (w469:T1)
      }
      frame "157" {
        n261 = shared-variable "RT Single-Board RIO\\Email Handler.lvlib\\Warning157"() -> (w472:bool)  [unwired: 1 in, 1 out]
        n262 = shared-variable "RT Single-Board RIO\\Email Handler.lvlib\\Inform157"() -> (w473:string)  [unwired: 1 in, 1 out]
        n263 = shared-variable "My Computer\\Email Handler.lvlib\\Email157"() -> (w474:string[])  [unwired: 1 in, 1 out]
        n264 = Bundle By Name(cluster=w476, "EmailArray"=w474, "Inform"=w473, "Alarm"=w472) -> (w475:T1)
      }
      frame "158" {
        n265 = shared-variable "RT Single-Board RIO\\Email Handler.lvlib\\Warning158"() -> (w478:bool)  [unwired: 1 in, 1 out]
        n266 = shared-variable "RT Single-Board RIO\\Email Handler.lvlib\\Inform158"() -> (w479:string)  [unwired: 1 in, 1 out]
        n267 = shared-variable "My Computer\\Email Handler.lvlib\\Email158"() -> (w480:string[])  [unwired: 1 in, 1 out]
        n268 = Bundle By Name(cluster=w482, "EmailArray"=w480, "Inform"=w479, "Alarm"=w478) -> (w481:T1)
      }
      frame "159" {
        n269 = shared-variable "RT Single-Board RIO\\Email Handler.lvlib\\Warning159"() -> (w484:bool)  [unwired: 1 in, 1 out]
        n270 = shared-variable "RT Single-Board RIO\\Email Handler.lvlib\\Inform159"() -> (w485:string)  [unwired: 1 in, 1 out]
        n271 = shared-variable "My Computer\\Email Handler.lvlib\\Email159"() -> (w486:string[])  [unwired: 1 in, 1 out]
        n272 = Bundle By Name(cluster=w488, "EmailArray"=w486, "Inform"=w485, "Alarm"=w484) -> (w487:T1)
      }
      frame "160" {
        n273 = shared-variable "RT Single-Board RIO\\Email Handler.lvlib\\Warning160"() -> (w490:bool)  [unwired: 1 in, 1 out]
        n274 = shared-variable "RT Single-Board RIO\\Email Handler.lvlib\\Inform160"() -> (w491:string)  [unwired: 1 in, 1 out]
        n275 = shared-variable "My Computer\\Email Handler.lvlib\\Email160"() -> (w492:string[])  [unwired: 1 in, 1 out]
        n276 = Bundle By Name(cluster=w494, "EmailArray"=w492, "Inform"=w491, "Alarm"=w490) -> (w493:T1)
      }
      frame "161" {
        n277 = shared-variable "RT Single-Board RIO\\Email Handler.lvlib\\Warning161"() -> (w496:bool)  [unwired: 1 in, 1 out]
        n278 = shared-variable "RT Single-Board RIO\\Email Handler.lvlib\\Inform161"() -> (w497:string)  [unwired: 1 in, 1 out]
        n279 = shared-variable "My Computer\\Email Handler.lvlib\\Email161"() -> (w498:string[])  [unwired: 1 in, 1 out]
        n280 = Bundle By Name(cluster=w500, "EmailArray"=w498, "Inform"=w497, "Alarm"=w496) -> (w499:T1)
      }
      frame "162" {
        n281 = shared-variable "RT Single-Board RIO\\Email Handler.lvlib\\Warning162"() -> (w502:bool)  [unwired: 1 in, 1 out]
        n282 = shared-variable "RT Single-Board RIO\\Email Handler.lvlib\\Inform162"() -> (w503:string)  [unwired: 1 in, 1 out]
        n283 = shared-variable "My Computer\\Email Handler.lvlib\\Email162"() -> (w504:string[])  [unwired: 1 in, 1 out]
        n284 = Bundle By Name(cluster=w506, "EmailArray"=w504, "Inform"=w503, "Alarm"=w502) -> (w505:T1)
      }
      frame "163" {
        n285 = shared-variable "RT Single-Board RIO\\Email Handler.lvlib\\Warning163"() -> (w508:bool)  [unwired: 1 in, 1 out]
        n286 = shared-variable "RT Single-Board RIO\\Email Handler.lvlib\\Inform163"() -> (w509:string)  [unwired: 1 in, 1 out]
        n287 = shared-variable "My Computer\\Email Handler.lvlib\\Email163"() -> (w510:string[])  [unwired: 1 in, 1 out]
        n288 = Bundle By Name(cluster=w512, "EmailArray"=w510, "Inform"=w509, "Alarm"=w508) -> (w511:T1)
      }
      frame "164" {
        n289 = shared-variable "RT Single-Board RIO\\Email Handler.lvlib\\Warning164"() -> (w514:bool)  [unwired: 1 in, 1 out]
        n290 = shared-variable "RT Single-Board RIO\\Email Handler.lvlib\\Inform164"() -> (w515:string)  [unwired: 1 in, 1 out]
        n291 = shared-variable "My Computer\\Email Handler.lvlib\\Email164"() -> (w516:string[])  [unwired: 1 in, 1 out]
        n292 = Bundle By Name(cluster=w518, "EmailArray"=w516, "Inform"=w515, "Alarm"=w514) -> (w517:T1)
      }
      frame "165" {
        n293 = shared-variable "RT Single-Board RIO\\Email Handler.lvlib\\Warning165"() -> (w520:bool)  [unwired: 1 in, 1 out]
        n294 = shared-variable "RT Single-Board RIO\\Email Handler.lvlib\\Inform165"() -> (w521:string)  [unwired: 1 in, 1 out]
        n295 = shared-variable "My Computer\\Email Handler.lvlib\\Email165"() -> (w522:string[])  [unwired: 1 in, 1 out]
        n296 = Bundle By Name(cluster=w524, "EmailArray"=w522, "Inform"=w521, "Alarm"=w520) -> (w523:T1)
      }
      frame "166" {
        n297 = shared-variable "RT Single-Board RIO\\Email Handler.lvlib\\Warning166"() -> (w526:bool)  [unwired: 1 in, 1 out]
        n298 = shared-variable "RT Single-Board RIO\\Email Handler.lvlib\\Inform166"() -> (w527:string)  [unwired: 1 in, 1 out]
        n299 = shared-variable "My Computer\\Email Handler.lvlib\\Email166"() -> (w528:string[])  [unwired: 1 in, 1 out]
        n300 = Bundle By Name(cluster=w530, "EmailArray"=w528, "Inform"=w527, "Alarm"=w526) -> (w529:T1)
      }
      frame "167" {
        n301 = shared-variable "RT Single-Board RIO\\Email Handler.lvlib\\Warning167"() -> (w532:bool)  [unwired: 1 in, 1 out]
        n302 = shared-variable "RT Single-Board RIO\\Email Handler.lvlib\\Inform167"() -> (w533:string)  [unwired: 1 in, 1 out]
        n303 = shared-variable "My Computer\\Email Handler.lvlib\\Email167"() -> (w534:string[])  [unwired: 1 in, 1 out]
        n304 = Bundle By Name(cluster=w536, "EmailArray"=w534, "Inform"=w533, "Alarm"=w532) -> (w535:T1)
      }
      frame "168" {
        n305 = shared-variable "RT Single-Board RIO\\Email Handler.lvlib\\Warning168"() -> (w538:bool)  [unwired: 1 in, 1 out]
        n306 = shared-variable "RT Single-Board RIO\\Email Handler.lvlib\\Inform168"() -> (w539:string)  [unwired: 1 in, 1 out]
        n307 = shared-variable "My Computer\\Email Handler.lvlib\\Email168"() -> (w540:string[])  [unwired: 1 in, 1 out]
        n308 = Bundle By Name(cluster=w542, "EmailArray"=w540, "Inform"=w539, "Alarm"=w538) -> (w541:T1)
      }
      frame "169" {
        n309 = shared-variable "RT Single-Board RIO\\Email Handler.lvlib\\Warning169"() -> (w544:bool)  [unwired: 1 in, 1 out]
        n310 = shared-variable "RT Single-Board RIO\\Email Handler.lvlib\\Inform169"() -> (w545:string)  [unwired: 1 in, 1 out]
        n311 = shared-variable "My Computer\\Email Handler.lvlib\\Email169"() -> (w546:string[])  [unwired: 1 in, 1 out]
        n312 = Bundle By Name(cluster=w548, "EmailArray"=w546, "Inform"=w545, "Alarm"=w544) -> (w547:T1)
      }
      frame "170" {
        n313 = shared-variable "RT Single-Board RIO\\Email Handler.lvlib\\Warning170"() -> (w550:bool)  [unwired: 1 in, 1 out]
        n314 = shared-variable "RT Single-Board RIO\\Email Handler.lvlib\\Inform170"() -> (w551:string)  [unwired: 1 in, 1 out]
        n315 = shared-variable "My Computer\\Email Handler.lvlib\\Email170"() -> (w552:string[])  [unwired: 1 in, 1 out]
        n316 = Bundle By Name(cluster=w554, "EmailArray"=w552, "Inform"=w551, "Alarm"=w550) -> (w553:T1)
      }
      frame "171" {
        n317 = shared-variable "RT Single-Board RIO\\Email Handler.lvlib\\Warning171"() -> (w556:bool)  [unwired: 1 in, 1 out]
        n318 = shared-variable "RT Single-Board RIO\\Email Handler.lvlib\\Inform171"() -> (w557:string)  [unwired: 1 in, 1 out]
        n319 = shared-variable "My Computer\\Email Handler.lvlib\\Email171"() -> (w558:string[])  [unwired: 1 in, 1 out]
        n320 = Bundle By Name(cluster=w560, "EmailArray"=w558, "Inform"=w557, "Alarm"=w556) -> (w559:T1)
      }
      frame "172" {
        n321 = shared-variable "RT Single-Board RIO\\Email Handler.lvlib\\Warning172"() -> (w562:bool)  [unwired: 1 in, 1 out]
        n322 = shared-variable "RT Single-Board RIO\\Email Handler.lvlib\\Inform172"() -> (w563:string)  [unwired: 1 in, 1 out]
        n323 = shared-variable "My Computer\\Email Handler.lvlib\\Email172"() -> (w564:string[])  [unwired: 1 in, 1 out]
        n324 = Bundle By Name(cluster=w566, "EmailArray"=w564, "Inform"=w563, "Alarm"=w562) -> (w565:T1)
      }
      frame "173" {
        n325 = shared-variable "RT Single-Board RIO\\Email Handler.lvlib\\Warning173"() -> (w568:bool)  [unwired: 1 in, 1 out]
        n326 = shared-variable "RT Single-Board RIO\\Email Handler.lvlib\\Inform173"() -> (w569:string)  [unwired: 1 in, 1 out]
        n327 = shared-variable "My Computer\\Email Handler.lvlib\\Email173"() -> (w570:string[])  [unwired: 1 in, 1 out]
        n328 = Bundle By Name(cluster=w572, "EmailArray"=w570, "Inform"=w569, "Alarm"=w568) -> (w571:T1)
      }
      frame "174" {
        n329 = shared-variable "RT Single-Board RIO\\Email Handler.lvlib\\Warning174"() -> (w574:bool)  [unwired: 1 in, 1 out]
        n330 = shared-variable "RT Single-Board RIO\\Email Handler.lvlib\\Inform174"() -> (w575:string)  [unwired: 1 in, 1 out]
        n331 = shared-variable "My Computer\\Email Handler.lvlib\\Email174"() -> (w576:string[])  [unwired: 1 in, 1 out]
        n332 = Bundle By Name(cluster=w578, "EmailArray"=w576, "Inform"=w575, "Alarm"=w574) -> (w577:T1)
      }
      frame "175" {
        n333 = shared-variable "RT Single-Board RIO\\Email Handler.lvlib\\Warning175"() -> (w580:bool)  [unwired: 1 in, 1 out]
        n334 = shared-variable "RT Single-Board RIO\\Email Handler.lvlib\\Inform175"() -> (w581:string)  [unwired: 1 in, 1 out]
        n335 = shared-variable "My Computer\\Email Handler.lvlib\\Email175"() -> (w582:string[])  [unwired: 1 in, 1 out]
        n336 = Bundle By Name(cluster=w584, "EmailArray"=w582, "Inform"=w581, "Alarm"=w580) -> (w583:T1)
      }
    }
  }
